vi "Handle UNSUBSCRIBED.vi"(8 "error in (no error)":errorcluster, 9 "Unsubscribe Reqeusts (in)":T1, 10 "WAMP Message":T14 {"Message Codes" items=["HELLO"=1, "WELCOME"=2, "ABORT"=3, "GOODBYE"=6, "ERROR"=8, "PUBLISH"=16, "PUBLISHED"=17, "SUBSCRIBE"=32, "SUBSCRIBED"=33, "UNSUBSCRIBE"=34, "UNSUBSCRIBED"=35, "EVENT"=36, "CALL"=48, "RESULT"=59, "REGISTER"=64, "REGISTERED"=65, "UNREGISTER"=66, "UNREGISTERED"=67, "INVOCATION"=68, "YIELD"=70]}, 11 "reference":refnum<class "WAMP Client.lvclass">) -> (0 "error out":errorcluster, 1 "Message Loop Data (Out)":T1, 3 "reference out":refnum<class "WAMP Client.lvclass">)   [LabVIEW 2020, in "wamplv.lvlib" / "WAMP Client.lvclass"]
uses:
  <userlib>/wamplv/WAMP Client/WAMP Client.lvclass
  <userlib>/wamplv/WAMP Client/TypeDef/WAMP Received Message.ctl
  <userlib>/wamplv/WAMP Message Codes.ctl
  <userlib>/wamplv/WAMP Client/TypeDef/Message Loop Shift Reg Data.ctl
  <userlib>/wamplv/WAMP Client/TypeDef/REGISTER Request Data.ctl
  <userlib>/wamplv/WAMP Client/TypeDef/REGISTERED or ERROR payload.ctl
  <userlib>/wamplv/WAMP Client/TypeDef/WAMP Error Payload.ctl
  <userlib>/wamplv/WAMP Client/TypeDef/INVOCATION payload.ctl
  <userlib>/wamplv/WAMP Client/TypeDef/Publish Requests Map.ctl
  <userlib>/wamplv/WAMP Client/TypeDef/PUBLISH Request Data.ctl
  <userlib>/wamplv/WAMP Client/TypeDef/PUBLISH Result.ctl
  <userlib>/wamplv/WAMP Client/TypeDef/Endpoint Data.ctl
  <userlib>/wamplv/WAMP Client/TypeDef/CALL Request Map.ctl
  <userlib>/wamplv/WAMP Client/TypeDef/CALL Request Data.ctl
  <userlib>/wamplv/WAMP Client/TypeDef/RESULT Payload.ctl
  <userlib>/wamplv/WAMP Client/TypeDef/SUBSCRIBE Requests Map.ctl
  <userlib>/wamplv/WAMP Client/TypeDef/SUBSCRIBE Request Data.ctl
  <userlib>/wamplv/WAMP Client/TypeDef/Subscribe Result.ctl
  <userlib>/wamplv/WAMP Client/TypeDef/Event Payload.ctl
  <userlib>/wamplv/WAMP Client/TypeDef/Subscriptions Map.ctl
  <userlib>/wamplv/WAMP Client/TypeDef/Subscription Details.ctl
  <userlib>/wamplv/WAMP Client/TypeDef/Unsubscribe Requests Map.ctl
  <userlib>/wamplv/WAMP Client/TypeDef/UNSUBSCRIBE Request Data.ctl
  <userlib>/wamplv/WAMP Client/TypeDef/UNSUBSCRIBE Result.ctl
  <userlib>/wamplv/WAMP Client/WAMP Client.lvclass/WAMP Client.ctl
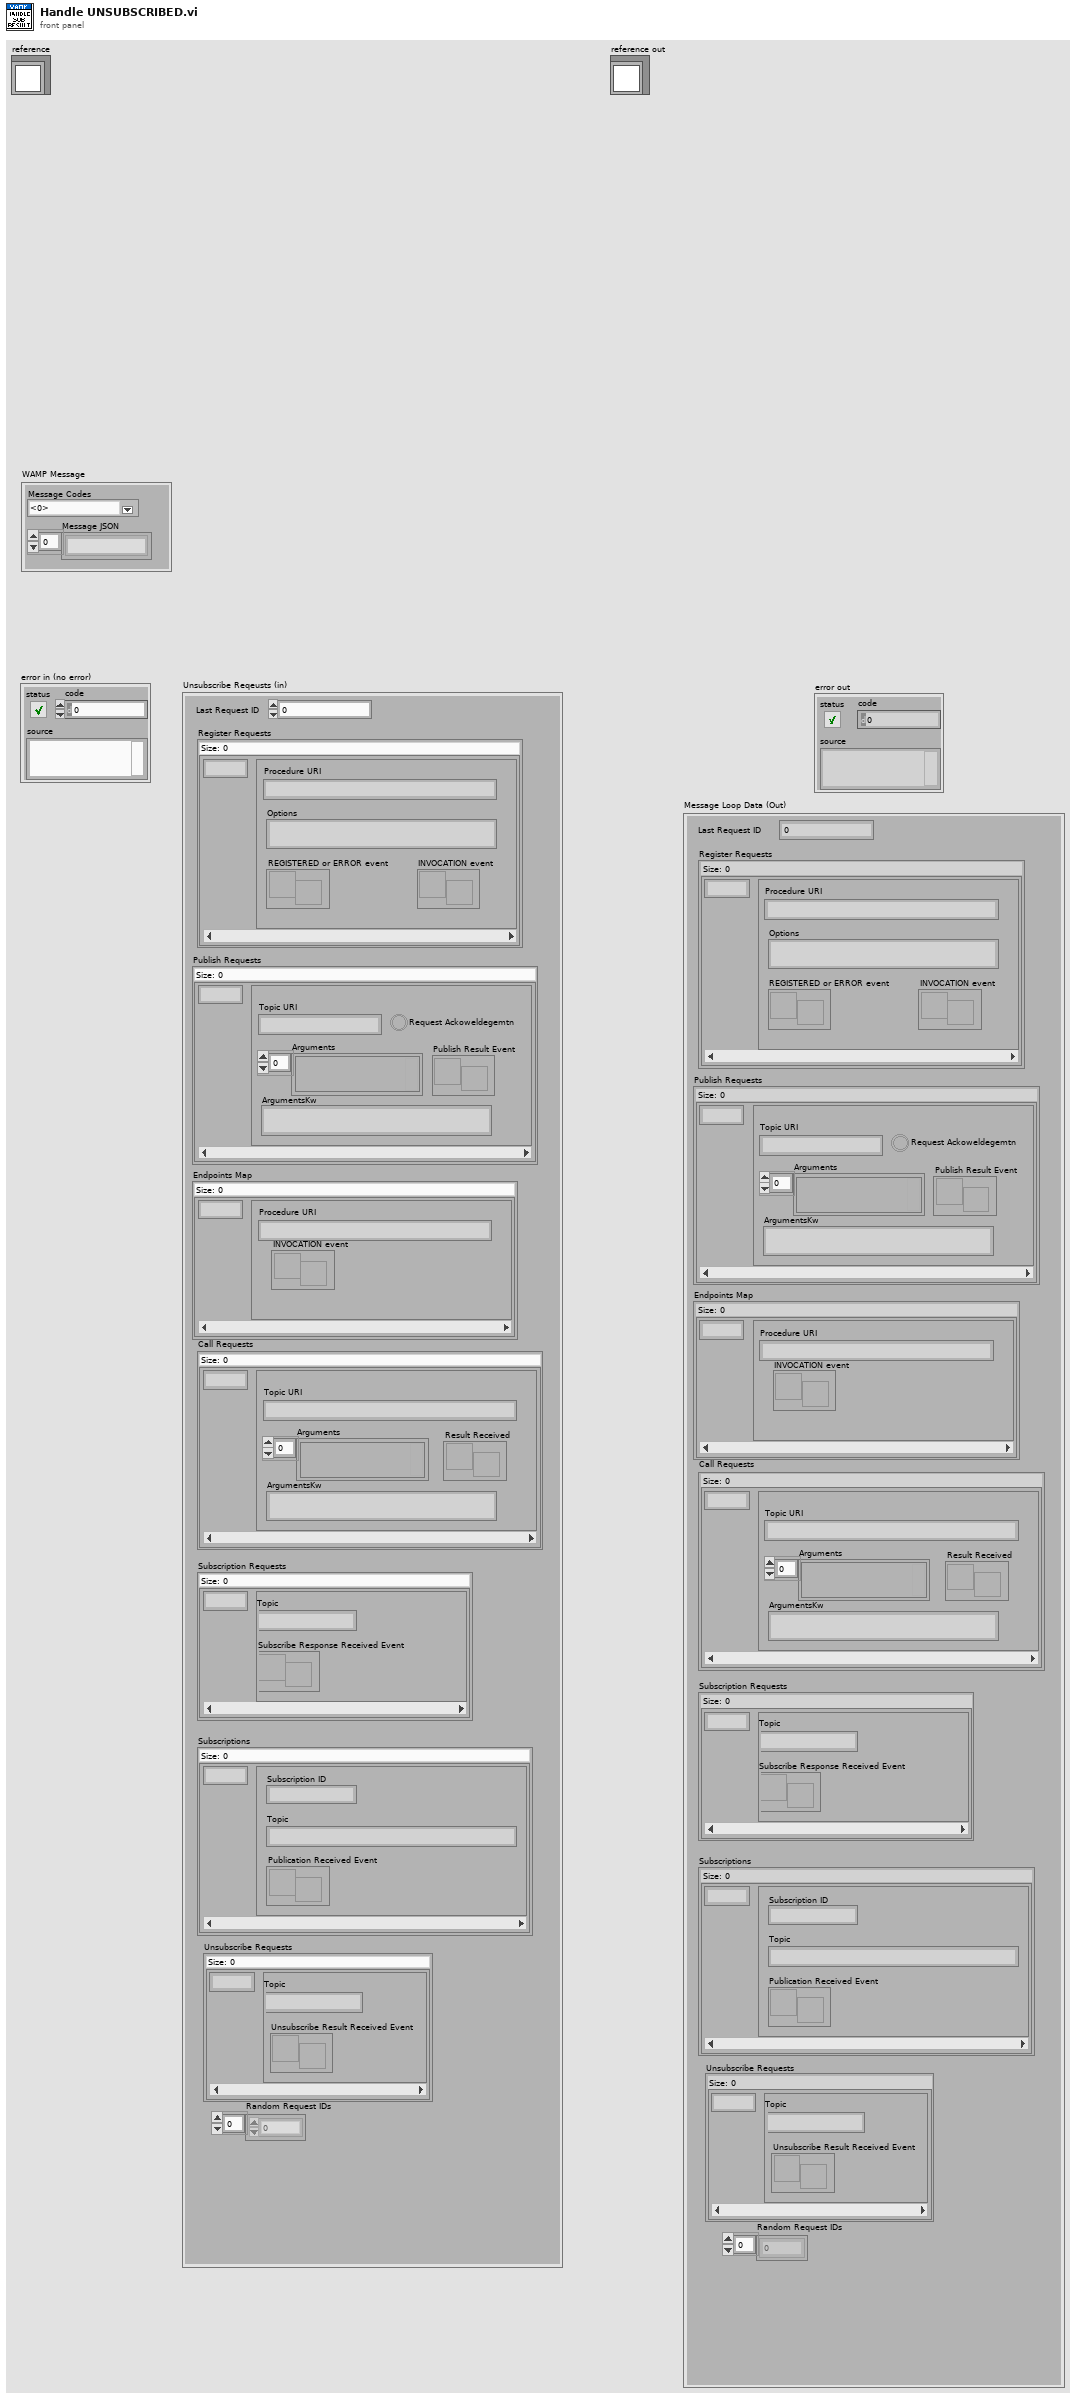
[diagram p1: front panel]
types:
  T1 = typedef "wamplv.lvlib/WAMP Client.lvclass/Message Loop Shift Reg Data.ctl" = cluster{"Last Request ID":u64, "Register Requests":map{u64, T2}, "Publish Requests":T3, "Endpoints Map":map{u64, T5}, "Call Requests":T6, "Subscription Requests":T8, "Subscriptions":T10, "Unsubscribe Requests":T12, "Random Request IDs":u64[]}
  T2 = typedef "wamplv.lvlib/WAMP Client.lvclass/REGISTER Request Data.ctl" = cluster{"Procedure URI":string, "Options":string, "REGISTERED or ERROR event":refnum<user-event>, "INVOCATION event":refnum<user-event>}
  T3 = typedef "wamplv.lvlib/WAMP Client.lvclass/Publish Requests Map.ctl" = map{u64, T4}
  T4 = typedef "wamplv.lvlib/WAMP Client.lvclass/PUBLISH Request Data.ctl" = cluster{"Topic URI":string, "Arguments":variant[], "ArgumentsKw":string, "Publish Result Event":refnum<user-event>, "Request Ackoweldegemtn":bool}
  T5 = typedef "wamplv.lvlib/WAMP Client.lvclass/Endpoint Data.ctl" = cluster{"Procedure URI":string, "INVOCATION event":refnum<user-event>}
  T6 = typedef "wamplv.lvlib/WAMP Client.lvclass/CALL Request Map.ctl" = map{u64, T7}
  T7 = typedef "wamplv.lvlib/WAMP Client.lvclass/CALL Request Data.ctl" = cluster{"Topic URI":string, "Arguments":variant[], "ArgumentsKw":string, "Result Received":refnum<user-event>}
  T8 = typedef "wamplv.lvlib/WAMP Client.lvclass/SUBSCRIBE Requests Map.ctl" = map{u64, T9}
  T9 = typedef "wamplv.lvlib/WAMP Client.lvclass/SUBSCRIBE Request Data.ctl" = cluster{"Topic":string, "Subscribe Response Received Event":refnum<user-event>}
  T10 = typedef "wamplv.lvlib/WAMP Client.lvclass/Subscriptions Map.ctl" = map{u64, T11}
  T11 = typedef "wamplv.lvlib/WAMP Client.lvclass/Subscription Details.ctl" = cluster{"Subscription ID":u64, "Topic":string, "Publication Received Event":refnum<user-event>}
  T12 = typedef "wamplv.lvlib/WAMP Client.lvclass/Unsubscribe Requests Map.ctl" = map{u64, T13}
  T13 = typedef "wamplv.lvlib/WAMP Client.lvclass/UNSUBSCRIBE Request Data.ctl" = cluster{"Topic":string, "Unsubscribe Result Received Event":refnum<user-event>}
  T14 = typedef "wamplv.lvlib/WAMP Client.lvclass/WAMP Received Message.ctl" = cluster{"Message JSON":string[], "Message Codes":T15}
  T15 = typedef "wamplv.lvlib/WAMP Client.lvclass/WAMP Message Codes.ctl" = u16
  T16 = typedef "wamplv.lvlib/WAMP Client.lvclass/UNSUBSCRIBE Result.ctl" = cluster{"Success?":bool, "Error":errorcluster}
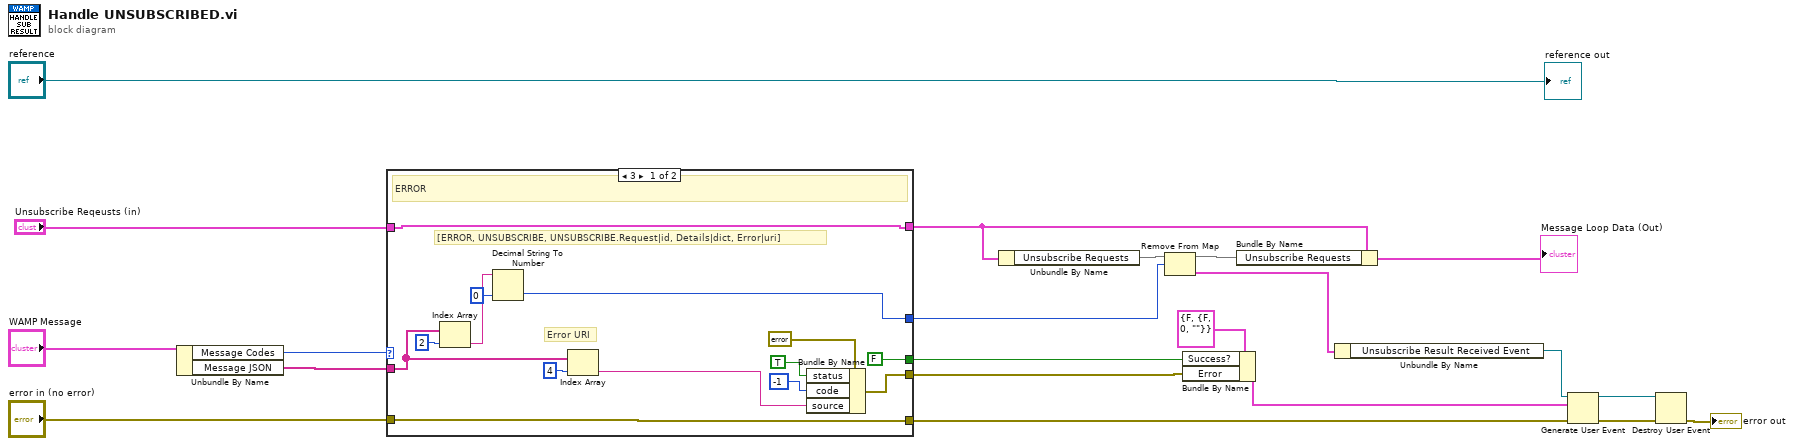
[diagram p0: block diagram]
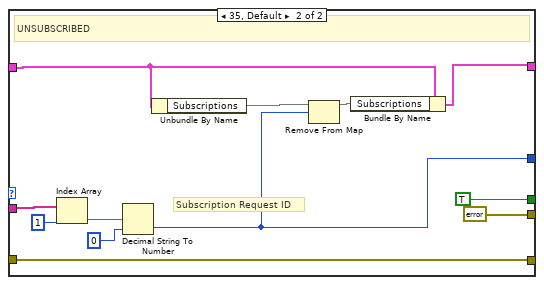
[diagram p2: hidden frame]
diagram:
  n1 = Unbundle By Name("WAMP Message") -> ("Message Codes"=w14:T15, "Message JSON"=w13:string[])
  n2 = case shown="3" w14 {
    tunnel: w13 -> [w33 w46]
    tunnel: [w24 w40] -> w12
    tunnel: "error in (no error)" -> [w27 w45]
    tunnel: [w27 w45] -> w17
    tunnel: [w28 errorcluster {"status"=FALSE, "code"=0, "source"=""} ("error in (no error)")] -> w20
    tunnel: [FALSE ("Success?") TRUE ("Success?")] -> w19
    tunnel: "Unsubscribe Reqeusts (in)" -> [w23 w37]
    tunnel: [w23 w36] -> w1
    frame 3 {
      # "Error URI"
      # "[ERROR, UNSUBSCRIBE, UNSUBSCRIBE.Request|id, Details|dict, Error|uri]"
      # "ERROR"
      n3 = Index Array(array=w33, index=2) -> (element=w34:string)
      n4 = Decimal String To Number(string=w34, default (0L)=u64 0 ("default (0 I32)")) -> (number=w24:u64)  [unwired: 1 in, 1 out]
      n5 = Index Array(array=w33, index=4) -> (element=w30:string)
      n6 = Bundle By Name(cluster=errorcluster {"status"=FALSE, "code"=0, "source"=""} ("error in (no error)"), "status"=TRUE, "code"=-1, "source"=w30) -> (w28:errorcluster)
    }
    frame 35, Default {
      # "Subscription Request ID"
      # "UNSUBSCRIBED"
      n7 = Index Array(array=w46, index=1) -> (element=w42:string)
      n8 = Decimal String To Number(string=w42, default (0L)=u64 0) -> (number=w40:u64)  [unwired: 1 in, 1 out]
      n9 = Unbundle By Name(w37) -> ("Subscriptions"=w39:T10)
      n10 = Remove From Map(10:w40, 11:w39) -> (3:w38:T10)  [unwired: 2 out]
      n11 = Bundle By Name(cluster=w37, "Subscriptions"=w38) -> (w36:T1)
    }
  }
  n12 = Unbundle By Name(w1) -> ("Unsubscribe Requests"=w3:T12)
  n13 = Remove From Map(10:w12, 11:w3) -> (1:w11:T13, 3:w4:T12)  [unwired: 1 out]
  n14 = Bundle By Name(cluster=T16 {"Success?"=FALSE, "Error"={"status"=FALSE, "code"=0, "source"=""}} ("Unsubcsribe Result"), "Success?"=w19, "Error"=w20) -> (w18:T16)
  n15 = Bundle By Name(cluster=w1, "Unsubscribe Requests"=w4) -> (→"Message Loop Data (Out)":T1)
  n16 = Unbundle By Name(w11) -> ("Unsubscribe Result Received Event"=w6:refnum<user-event>)
  n17 = Generate User Event(user event=w6, event data cluster=w18, error in=w17) -> (user event out=w8:refnum<user-event>, error out=w10:errorcluster)  [unwired: 1 in]
  n18 = Destroy User Event(user event=w8, error in=w10) -> (error out=→"error out":errorcluster)
  "reference out" <- "reference"
